vi "N6701A_MonitorVoltageCurrent.vi"(4 "current lower limit":dbl, 5 "voltage lower limit":dbl, 6 "current upper limit":dbl, 7 "voltage upper limit":dbl, 8 "error in":errorcluster {"code" format="%.0x"}, 9 "Test Duration (s)":dbl, 10 "Channel Name (1)":string="1", 11 "VISA resource name":refnum<visa-resource-name>) -> (0 "error out":errorcluster, 1 "Current":dbl format="%^.3e", 2 "Voltage":dbl format="%^.3e", 3 "pass":bool)   [LabVIEW 2015]
uses:
  <instrlib>/Agilent N6700 Series/Agilent N6700 Series.lvlib
panel:
  out "Current Duration":dbl
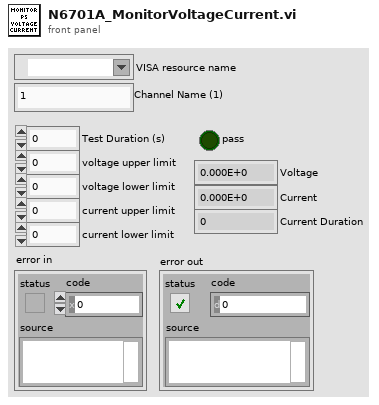
[diagram p1: front panel]
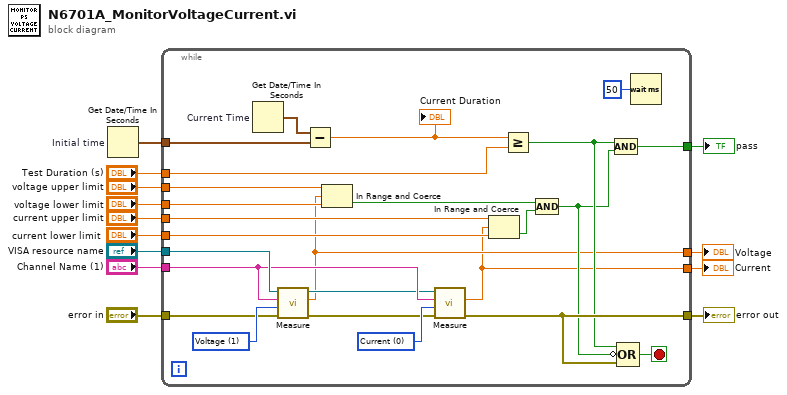
[diagram p0: block diagram]
diagram:
  n1 = Get Date/Time In Seconds "Initial time"() -> (seconds since 1Jan1904=w6:timestamp)
  n2 = while {
    tunnel: "VISA resource name" -> [w36]
    tunnel: "Channel Name (1)" -> [w35]
    tunnel: "error in" -> [w30]
    tunnel: [w29] -> w3
    tunnel: "voltage upper limit" -> [w27]
    tunnel: "voltage lower limit" -> [w26]
    tunnel: "current upper limit" -> [w25]
    tunnel: "current lower limit" -> [w24]
    tunnel: w6 -> [w22]
    tunnel: "Test Duration (s)" -> [w20]
    tunnel: [w17] -> w4
    tunnel: [w16] -> w2
    tunnel: [w15] -> w1
    stop <- w28 stop-if-true
    w37 = 0 items=["Voltage"=1, "Current"=0] ("Measurement Type (1: Voltage)")
    w38 = 1 items=["Voltage"=1, "Current"=0] ("Measurement Type (1: Voltage)")
    n3 = Get Date/Time In Seconds "Current Time"() -> (seconds since 1Jan1904=w23:timestamp)
    n4 = call <instrlib>:"Measure.vi"("error in (no error)"=w30, "Measurement Type (1: Voltage)"=w38, "Channel Name (1)"=w35, "VISA resource name"=w36) -> ("error out"=w34:errorcluster, "Measurement"=w16:dbl, "VISA resource name out"=w33:refnum<visa-resource-name>)  [unwired: 5 in]
    n5 = Subtract(x=w23, y=w22) -> (x-y=w21:dbl)
    "Current Duration" <- w21
    n6 = In Range and Coerce(upper limit=w27, x=w16, lower limit=w26) -> (In Range?=w31:bool)  [unwired: 1 out]
    n7 = call <instrlib>:"Measure.vi"("error in (no error)"=w34, "Measurement Type (1: Voltage)"=w37, "Channel Name (1)"=w35, "VISA resource name"=w33) -> ("error out"=w29:errorcluster, "Measurement"=w15:dbl)  [unwired: 5 in, 1 out]
    n8 = In Range and Coerce(upper limit=w25, x=w15, lower limit=w24) -> (In Range?=w32:bool)  [unwired: 1 out]
    n9 = Greater Or Equal?(x=w21, y=w20) -> (x >= y?=w19:bool)
    n10 = Compound Arithmetic op=AND(w31, w32) -> (w18:bool)
    n11 = Compound Arithmetic op=AND(w19, w18) -> (w17:bool)
    n12 = Compound Arithmetic op=OR(w19, invert w18, w29) -> (w28:bool)
    n13 = Wait (ms)(milliseconds to wait=u32 50) -> ()  [unwired: 1 out]
  }
  "pass" <- w4
  "error out" <- w3
  "Voltage" <- w2
  "Current" <- w1
